vi "PH_AxisGUI_BaseClass.CheckInterface.vi"(0 "i ref in":refnum<vi>, 5 "error in":errorcluster) -> (14 "i ref out":refnum<vi>, 19 "error out":errorcluster)   [LabVIEW 2014]
uses:
  PH_AxisGUI_6P/PH_AxisGUI_6P.lvlib
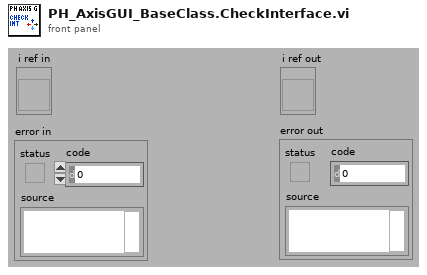
[diagram p1: front panel]
types:
  T1 = typedef "PH_AxisGUI_6P.lvlib/PH_AxisGUI_6P.i attribute.ctl" = cluster{"GUI Refs":T2, "Axis 1 Moving":bool, "Axis 2 Moving":bool, "Axis 1 State":T3, "Axis 2 State":T3}
  T2 = typedef "PH_AxisGUI_6P.lvlib/PH_AxisGUI_6P.GUI Refs.ctl" = cluster{"UP":refnum<vi>, "DOWN":refnum<vi>, "LEFT":refnum<vi>, "RIGHT":refnum<vi>, "Axis1_Status":refnum<vi>, "Axis2_Status":refnum<vi>, "Axis1_Target":refnum<vi>, "Axis2_Target":refnum<vi>, "Axis1_Address":refnum<vi>, "Axis2_Address":refnum<vi>, "Axis1_Advanced":refnum<vi>, "Axis2_Advanced":refnum<vi>, "AxisSelection":refnum<vi>, "Tab Control":refnum<vi>, "StopMotor":refnum<vi>, "SetZero":refnum<vi>, "Reset Controller":refnum<vi>, "Axis1_Status Bar":refnum<vi>, "Axis2_Status Bar":refnum<vi>, "Axis1_Settings":refnum<vi>, "Axis2_Settings":refnum<vi>}
  T3 = typedef "PH_Motion.Axis State.ctl" = enum16{"NoLink", "Inactive", "Active", "Error", "NoInfo"}
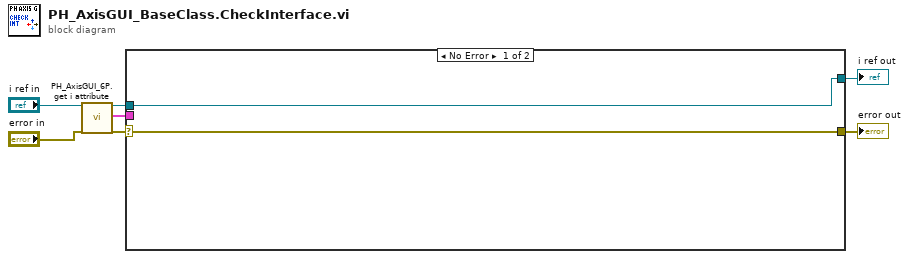
[diagram p0: block diagram]
diagram:
  n1 = call "PH_AxisGUI_6P.get i attribute.vi"("i ref in"="i ref in", "error in (no error)"="error in") -> ("i ref out"=w4:refnum<vi>, "i attribute"=w1:T1, "error out"=w2:errorcluster)  [unwired: 15 in]
  n2 = case shown="No Error" w2 {
    selector: w2 -> [w8 w11]
    tunnel: w4 -> [w9 w10]
    tunnel: [w9 w10] -> w7
    tunnel: [w8 w11] -> w6
    tunnel: w1 -> [_ _]
    frame No Error {
    }
    frame Error {
    }
  }
  "error out" <- w6
  "i ref out" <- w7
